vi "Logging.Start.vi"(8 "error in (no error)":errorcluster, 11 "Root Folder":path=path "C:/Users/john/Desktop") -> (0 "error out":errorcluster)   [LabVIEW 2018]
uses:
  <vilib>/Field R&D Services/Logger/Public/Controls/Configuration.ctl
  <vilib>/Field R&D Services/Logger/Logger.lvlib
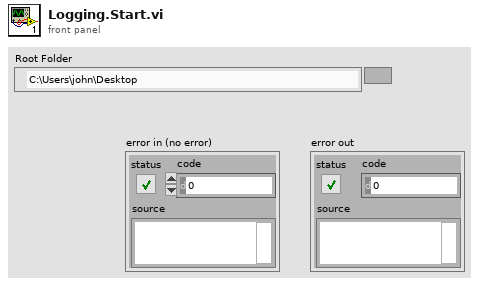
[diagram p1: front panel]
types:
  T1 = typedef "Logger.lvlib/Configuration.ctl" = cluster{"Root Folder":path, "Enable Calendar Tree":bool, "Maximum File Size":i64, "Maximum File Count":i32, "File Extension":string}
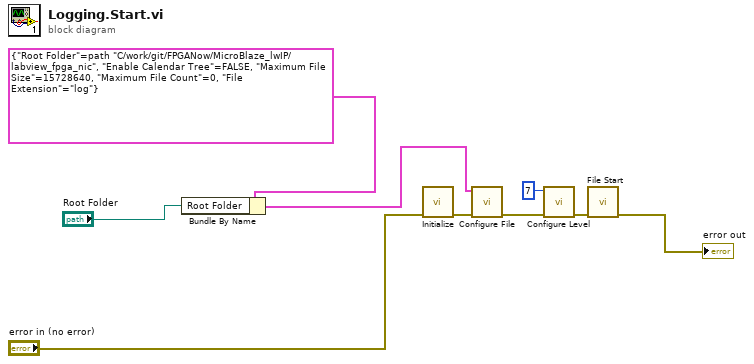
[diagram p0: block diagram]
diagram:
  n1 = Bundle By Name(cluster=T1 {"Root Folder"=path "C:/work/git/FPGANow/MicroBlaze_lwIP/labview_fpga_nic", "Enable Calendar Tree"=FALSE, "Maximum File Size"=15728640, "Maximum File Count"=0, "File Extension"="log"} ("Configuration"), "Root Folder"="Root Folder") -> (w1:T1)
  n2 = call <vilib>:"Initialize.vi"("Error In"="error in (no error)") -> ("Error Out"=w8:errorcluster)  [unwired: 10 in]
  n3 = call <vilib>:"Configure File.vi"("Error In"=w8, "Configuration"=w1) -> ("Error Out"=w9:errorcluster)  [unwired: 9 in]
  n4 = call <vilib>:"Configure Level.vi"("Error In"=w9, "Level"=u8 7) -> ("Error Out"=w7:errorcluster)  [unwired: 9 in]
  n5 = call <vilib>:"File Start.vi"("Error In"=w7) -> ("Error Out"=→"error out":errorcluster)  [unwired: 10 in]
